vi "Initialize.vi"(8 "error in":errorcluster, 10 "parameters":variant, 11 "CEF_Serialize node in":refnum<class "CEF_serializable node.lvclass">) -> (0 "error out":errorcluster, 2 "summary":T2[](array[typedef]), 3 "data value reference":T1)   [LabVIEW 2023, in "CEF.lvlib" / "CEF_serializable node.lvclass"]
doc: "Initializes the data of a node to its default state.\nThe object is not created inside of this VI, because it is created from a File depending on user selection.\nCopyright 2017 National Instruments Corporation\n\nLicensed under the Apache License, Version 2.0 (the \"License\"); you may not use this file except in compliance with the License. You may obtain a copy of the License at http://www.apache.org/licenses/LICENSE-2.0\nUnless required by applicable law or agreed to in writing, software distributed under the License is distributed on an \"AS IS\" BASIS, WITHOUT WARRANTIES OR CONDITIONS OF ANY KIND, either express or implied. See the License for the specific language governing permissions and limitations under the License."
uses:
  CEF_serializable node.lvclass
  Node/Summary.ctl
  Node/NodeRef.ctl
  Node/CEF_Node.lvclass
  serializable configuration/CEF_serializable configuration.lvclass
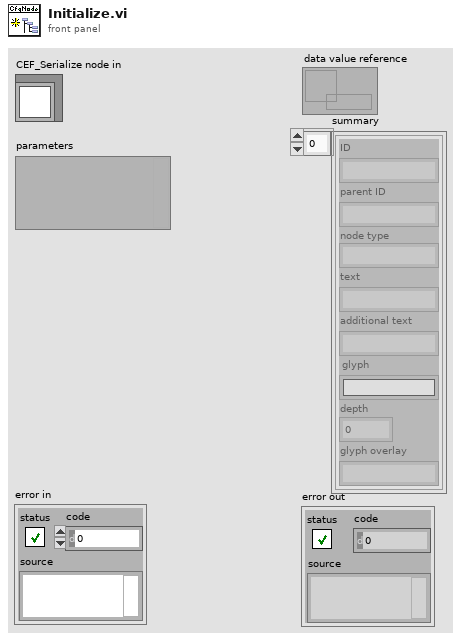
[diagram p1: front panel]
types:
  T1 = typedef "CEF.lvlib/CEF_Node.lvclass/NodeRef.ctl" = refnum<data-value>
  T2 = typedef "CEF.lvlib/CEF_Node.lvclass/Summary.ctl" = cluster{"ID":string, "parent ID":string, "node type":string, "text":string, "additional text":string, "glyph":string, "depth":i32, "glyph overlay":string}
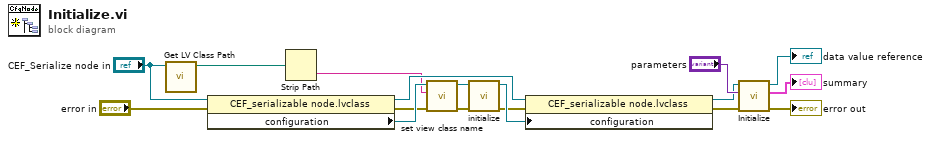
[diagram p0: block diagram]
diagram:
  n1 = call <vilib>:"Get LV Class Path.vi"("object"="CEF_Serialize node in") -> ("class path"=w2:path)  [unwired: 9 in, 1 out]
  n2 = property class="CEF_serializable node.lvclass"(reference="CEF_Serialize node in", error in="error in") -> (reference out=w10:refnum<class "CEF_serializable node.lvclass">, error out=w4:errorcluster, "configuration"=w7:refnum<class "CEF_serializable configuration.lvclass">)
  n3 = Strip Path(path=w2) -> (name=w1:string)  [unwired: 1 out]
  n4 = call "set view class name.vi"("error in"=w4, "view class"=w1, "CEF_Configuration in"=w7) -> ("error out"=w5:errorcluster, "CEF_Configuration out"=w6:refnum<class "CEF_serializable configuration.lvclass">)  [unwired: 7 in]
  n5 = call "initialize.vi"("error in"=w5, "CEF_Configuration in"=w6) -> ("error out"=w8:errorcluster, "CEF_Configuration out"=w9:refnum<class "CEF_serializable configuration.lvclass">)  [unwired: 7 in, 1 out]
  n6 = property class="CEF_serializable node.lvclass"(reference=w10, error in=w8, "configuration"=w9) -> (reference out=w11:refnum<class "CEF_serializable node.lvclass">, error out=w12:errorcluster)
  n7 = call-parent "Initialize.vi"("error in"=w12, "parameters"="parameters", "CEF_Node in"=w11) -> ("error out"=→"error out":errorcluster, "summary"=→"summary":T2[], "data value reference"=→"data value reference":T1)  [unwired: 6 in]
